vi "Motor_Ping_connect.vi"(8 "error in (no error)":errorcluster, 10 "remote port or service name":u16=7776, 11 "IP":string="192.168.24.142") -> (0 "error out":errorcluster, 1 "Connection Status":string, 2 "connection ID":refnum<k5>, 3 "ExitVI":bool)   [LabVIEW 2019]
panel:
  out "Received":string
  out "standard output":string
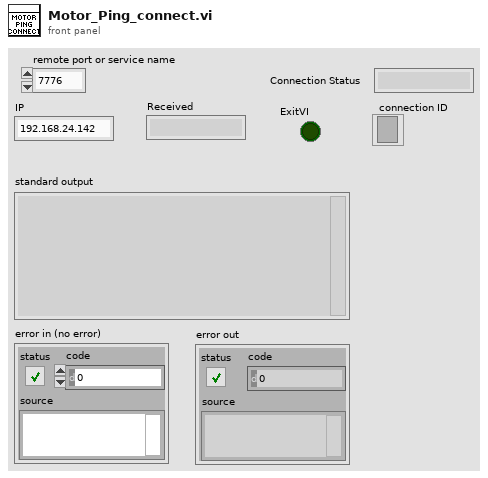
[diagram p1: front panel]
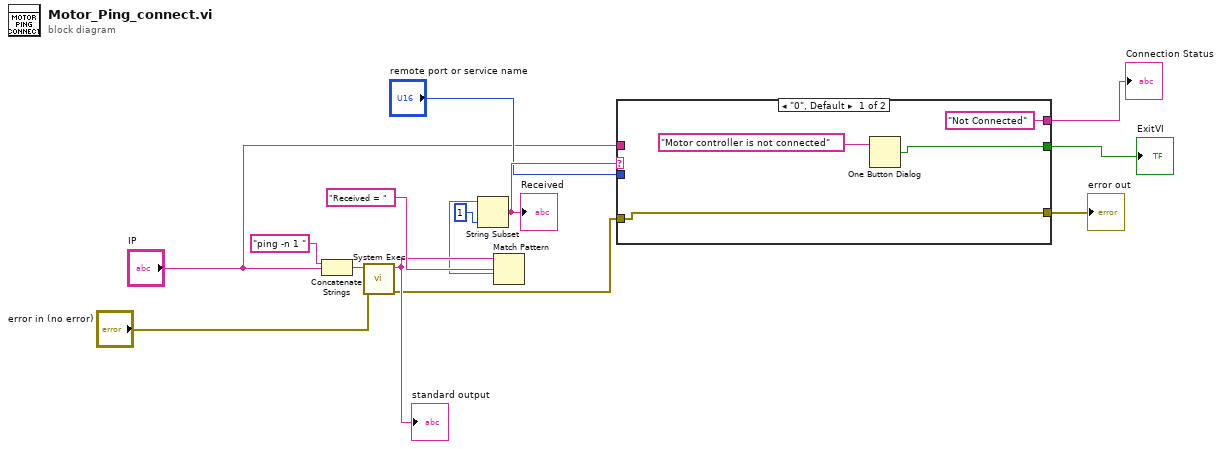
[diagram p0: block diagram]
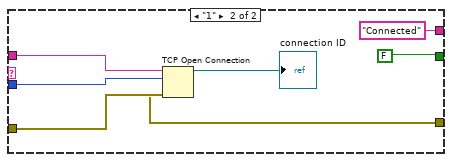
[diagram p2: hidden frame]
diagram:
  n1 = Concatenate Strings("ping -n 1 " ("string"), "IP") -> (w14:string)
  n2 = call <vilib>:"System Exec.vi"("error in (no error)"="error in (no error)", "command line"=w14) -> ("error out"=w2:errorcluster, "standard output"=w11:string)  [unwired: 6 in, 2 out]
  "standard output" <- w11
  n3 = Match Pattern(string=w11, regular expression="Received = ") -> (after substring=w10:string)  [unwired: 1 in, 3 out]
  n4 = String Subset(string=w10, length (rest)=1 ("length (rest)")) -> (substring=w8:string)  [unwired: 1 in]
  "Received" <- w8
  n5 = case shown="\"0\", Default" w8 {
    tunnel: [w16 FALSE ("T button?")] -> w7
    tunnel: "remote port or service name" -> [_ w24]
    tunnel: "IP" -> [_ w23]
    tunnel: [w18 w21] -> w3
    tunnel: w2 -> [w18 w22]
    tunnel: ["Not Connected" ("Connection Status") "Connected" ("Connection Status")] -> w1
    frame "0", Default {
      n6 = One Button Dialog(message="Motor controller is not connected") -> (true=w16:bool)  [unwired: 1 in]
    }
    frame "1" {
      n7 = TCP Open Connection(address=w23, remote port or service name=w24, error in (no error)=w22) -> (connection ID=→"connection ID":refnum<k5>, error out=w21:errorcluster)  [unwired: 2 in]
    }
  }
  "ExitVI" <- w7
  "error out" <- w3
  "Connection Status" <- w1
